vi "Finish Bleach.vi"(8 "error in (no error)":errorcluster, 11 "Application in":refnum<class "Application.lvclass">) -> (0 "error out":errorcluster, 3 "Application out":refnum<class "Application.lvclass">)   [LabVIEW 2018, in "Application.lvlib" / "Application.lvclass"]
uses:
  Application.lvclass
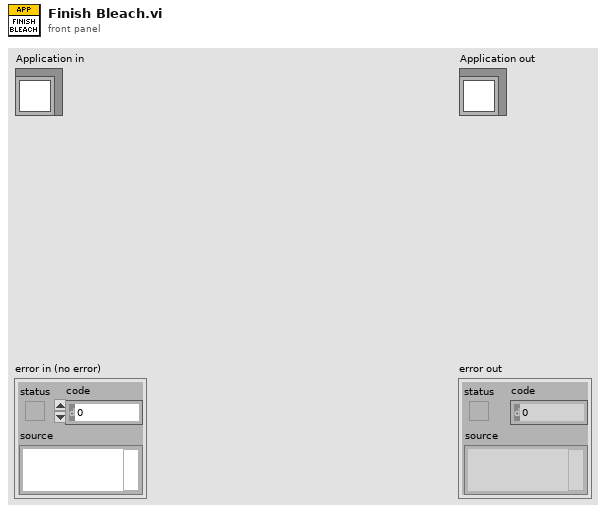
[diagram p1: front panel]
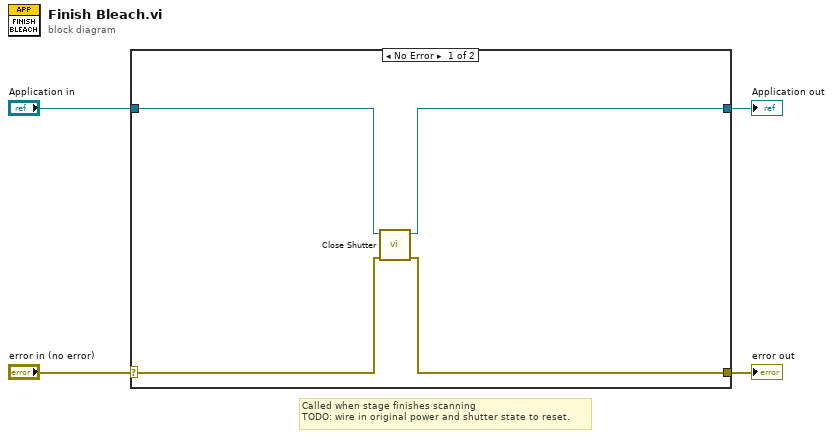
[diagram p0: block diagram]
diagram:
  # "Called when stage finishes scanning\nTODO: wire in original power and shutter state to reset."
  n1 = case shown="No Error" "error in (no error)" {
    selector: "error in (no error)" -> [w6 w10]
    tunnel: [w5 w10] -> w3
    tunnel: [w7 w9] -> w1
    tunnel: "Application in" -> [w8 w9]
    frame No Error {
      n2 = call-dynamic "Close Shutter.vi"("error in (no error)"=w6, "Application in"=w8) -> ("error out"=w5:errorcluster, "Application out"=w7:refnum<class "Application.lvclass">)  [unwired: 8 in]
    }
    frame Error {
    }
  }
  "error out" <- w3
  "Application out" <- w1
